vi "Add Pages.vi"(8 "error in (no error)":errorcluster) -> (0 "error out":errorcluster, 2 "latest data":T1)   [LabVIEW 2020, in "Rename As Application UI.lvlib" / "Configuration.lvlib"]
doc: "This VI adds all the different configuration views to the DCFG Framework as pages.\n\n_____\nBased on DCFG Project Template 1.0.0.21.\n____\nPeloton Config 1.0.0.2\nCopyright (c) 2022, Peloton"
uses:
  Configuration.lvlib
  Configuration--cluster.ctl
  Preferences UI.vi
  Settings UI.vi
  Configurations UI.vi
  <vilib>/Peloton/Peloton Config/Libraries/DCFG Framework/Peloton_DCFG Framework.lvlib
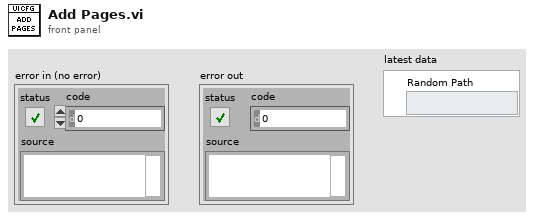
[diagram p1: front panel]
types:
  T1 = typedef "Rename As Application UI.lvlib/Configuration.lvlib/Configuration--cluster.ctl" = cluster{"Random Path":path}
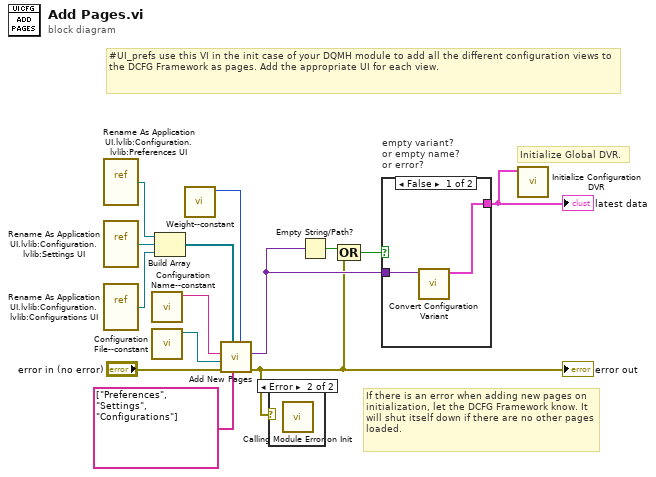
[diagram p0: block diagram]
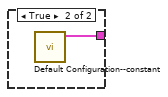
[diagram p3: hidden frame]
diagram:
  # "#UI_prefs use this VI in the init case of your DQMH module to add all the different configuration views to the DCFG Framework as pages. Add the appropriate UI for each view."
  # "If there is an error when adding new pages on initialization, let the DCFG Framework know. It will shut itself down if there are no other pages loaded."
  # "Initialize Global DVR."
  n1 = vi-ref "Rename As Application UI.lvlib:Configuration.lvlib:Preferences UI.vi"() -> (w11:refnum<vi>)
  n2 = vi-ref "Rename As Application UI.lvlib:Configuration.lvlib:Settings UI.vi"() -> (w13:refnum<vi>)
  n3 = vi-ref "Rename As Application UI.lvlib:Configuration.lvlib:Configurations UI.vi"() -> (w14:refnum<vi>)
  n4 = call "Configuration Name--constant.vi"() -> ("Configuration Name"=w8:string)  [unwired: 11 in]
  n5 = call "Configuration File--constant.vi"() -> ("Configuration File"=w10:refnum<class "Peloton_DCFG File.lvclass">)  [unwired: 11 in]
  n6 = Build Array(w11, w13, w14) -> (w12:refnum<vi>[])
  n7 = call "Weight--constant.vi"() -> ("Weight"=w1:i32)  [unwired: 11 in]
  n8 = call <vilib>:"Add New Pages.vi"("Weight"=w1, "Views"=string[] ["Preferences", "Settings", "Configurations"], "Pages"=w12, "error in (no error)"="error in (no error)", "Config File"=w10, "Page Name"=w8) -> ("error out"=w2:errorcluster, "Latest Data"=w7:variant)  [unwired: 4 in]
  "error out" <- w2
  n9 = case shown="Error" w2 {
    frame No Error {
    }
    frame Error {
      n10 = call <vilib>:"Calling Module Error on Init.vi"() -> ()  [unwired: 11 in, 1 out]
    }
  }
  n11 = Empty String/Path?(string/path=w7) -> (empty?=w6:bool)
  n12 = Compound Arithmetic op=OR(w6, w2) -> (w5:bool)
  n13 = case "empty variant?\nor empty name?\nor error?" shown="False" w5 {
    tunnel: [w15 w17] -> w4
    tunnel: w7 -> [w16 _]
    frame False {
      n14 = call "Convert Configuration Variant.vi"("Current Configuration"=w16) -> ("Configuration"=w15:T1)  [unwired: 8 in, 2 out]
    }
    frame True {
      n15 = call "Default Configuration--constant.vi"() -> ("Default Configuration"=w17:T1)  [unwired: 11 in]
    }
  }
  "latest data" <- w4
  n16 = call "Initialize Configuration DVR.vi"("Rename As Application UI Configuration"=w4) -> ()  [unwired: 11 in]
